vi "DAISY_polarity_signs.vi"(8 "Errors in":errorcluster[](array[cluster]), 11 "BoardHandles":T1(array[cluster])) -> (0 "Errors out":errorcluster[](array[cluster]), 2 "Polarity signs":dbl[](array[numeric]), 3 "BoardHandles Out":T1(array[cluster]))   [LabVIEW 2018]
uses:
  <instrlib>/CAEN PSM/CAEN PSM.lvlib
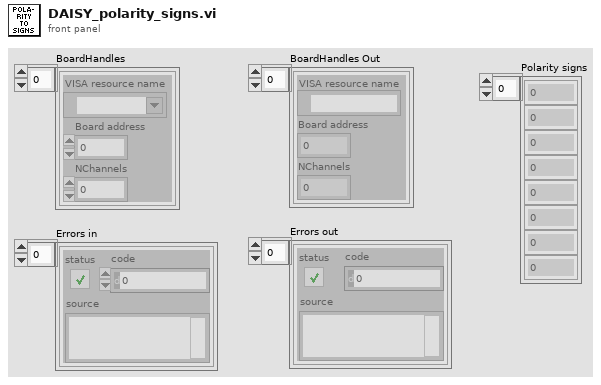
[diagram p1: front panel]
types:
  T1 = cluster{"VISA resource name":refnum<visa-resource-name>, "Board address":u8, "NChannels":u8}[]
  T2 = typedef "CAEN PSM.lvlib/BoardHandle.ctl" = cluster{"VISA resource name":refnum<visa-resource-name>, "Board address":u8, "NChannels":u8}
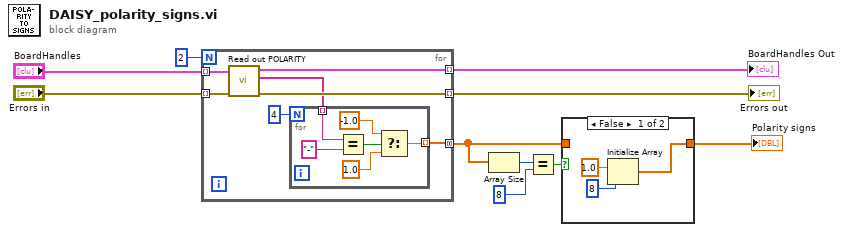
[diagram p0: block diagram]
diagram:
  n1 = for {
    N: 2 -> [_]
    tunnel: "BoardHandles" -> [w17] mode=indexing
    tunnel: "Errors in" -> [w16] mode=indexing
    tunnel: [w15] -> w4 mode=indexing
    tunnel: [w14] -> w5 mode=indexing
    tunnel: [w12] -> w9 mode=concatenating
    n2 = call <instrlib>:"Read out POLARITY.vi"("error in (no error)"=w16, "BoardHandle"=w17) -> ("error out"=w14:errorcluster, "Polarity values"=w13:string[], "BoardHandle out"=w15:T2)  [unwired: 7 in]
    n3 = for {
      N: 4 -> [_]
      tunnel: w13 -> [w22] mode=indexing
      tunnel: [w18] -> w12 mode=indexing
      n4 = Equal?(x=w22, y="-" ("Polarity value")) -> (x = y?=w21:bool)
      n5 = Select(t=-1.0, s=w21, f=1.0) -> (s? t:f=w18:dbl)
    }
  }
  "Errors out" <- w5
  "BoardHandles Out" <- w4
  n6 = Array Size(array=w9) -> (size(s)=w6:i32)
  n7 = Equal?(x=w6, y=8) -> (x = y?=w8:bool)
  n8 = case shown="False" w8 {
    tunnel: w9 -> [_ w27]
    tunnel: [w24 w27] -> w10
    frame False {
      n9 = Initialize Array(1.0 ("element"), 8 ("dimension size")) -> (w24:dbl[])
    }
    frame True {
    }
  }
  "Polarity signs" <- w10
